vi "자판기.vi"() -> ()   [LabVIEW 2023]
panel:
  in  "커피":bool
  in  "콜라":bool
  in  "아이스티":bool
  in  "반환":bool
  out "현재 금액":i32
  in  "종료":bool
  in  "물":bool
  in  "1000":bool
  in  "500":bool
  in  "100":bool
  # "커피"
  # "물"
  # "아이스티"
  # "콜라"
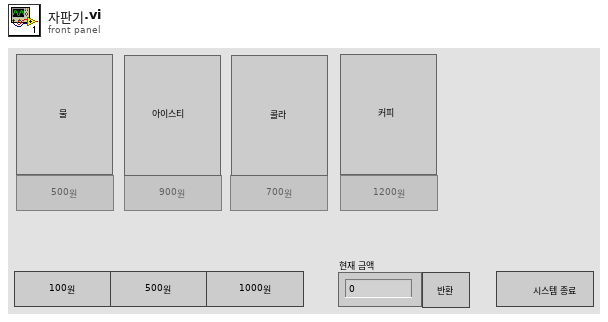
[diagram p1: front panel]
types:
  T1 = enum8{"Enabled", "Disabled", "Disabled and Grayed Out"}
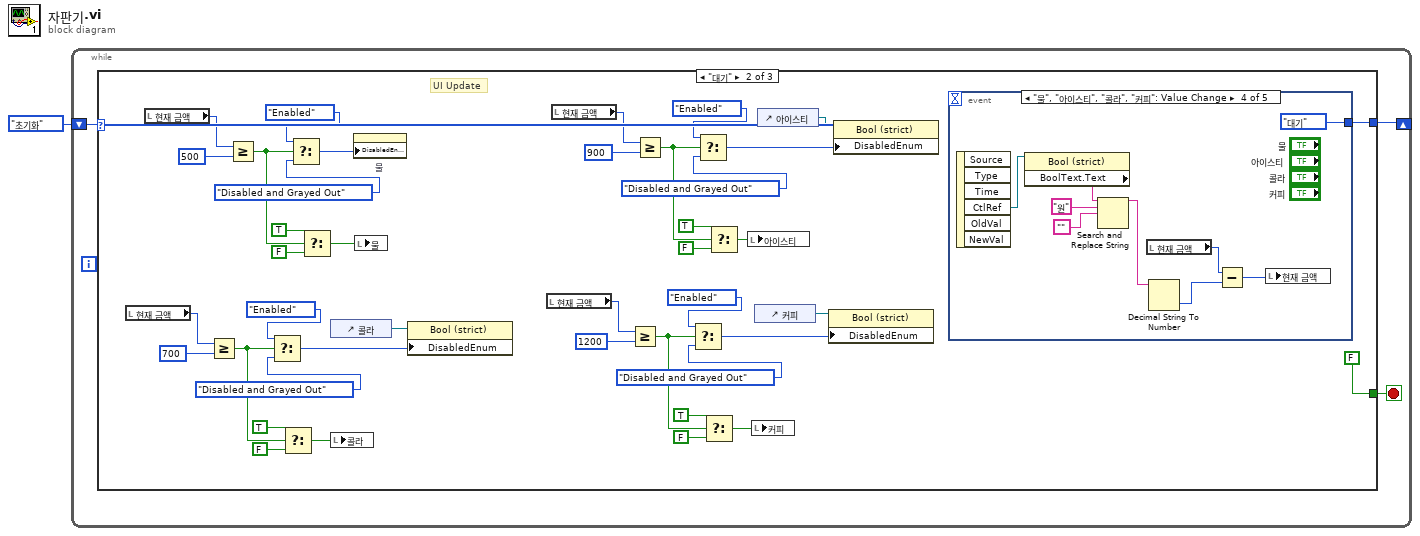
[diagram p0: block diagram]
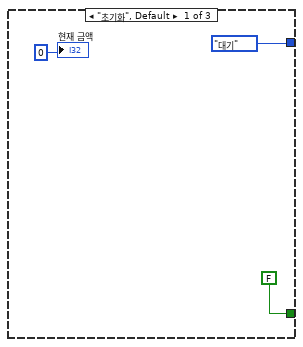
[diagram p2: hidden frame]
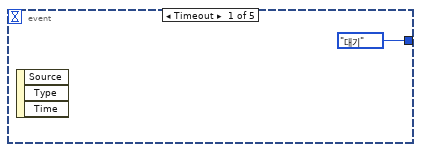
[diagram p3: hidden frame]
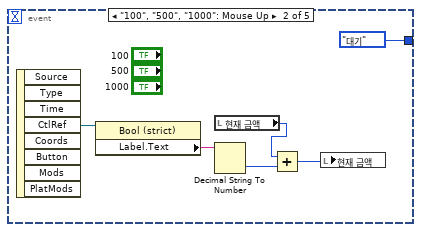
[diagram p4: hidden frame]
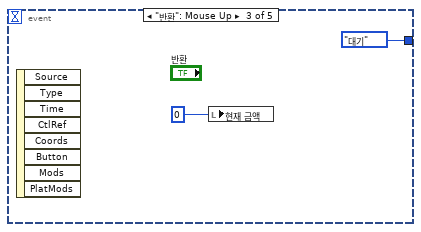
[diagram p5: hidden frame]
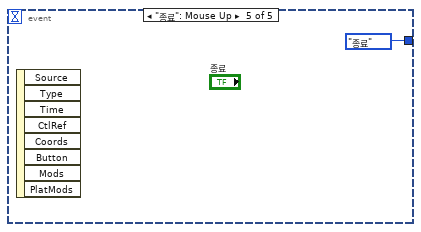
[diagram p6: hidden frame]
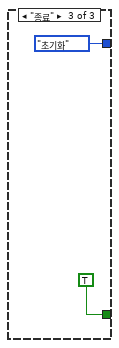
[diagram p7: hidden frame]
diagram:
  n1 = while {
    shift-right: [w3] -> _
    shift-left: enum16{"초기화", "대기", "종료"}."초기화" -> [w4]
    stop <- w2 stop-if-true
    n2 = case shown="\"대기\"" w4 {
      tunnel: [enum16{"초기화", "대기", "종료"}."대기" w48 enum16{"초기화", "대기", "종료"}."초기화"] -> w3
      tunnel: [FALSE FALSE TRUE] -> w2
      frame "초기화", Default {
        "현재 금액" <- 0 ("현재 금액")
      }
      frame "대기" {
        # "UI Update"
        n3 = local read "현재 금액"() -> (w28:i32)
        n4 = local read "현재 금액"() -> (w47:i32)
        n5 = Greater Or Equal?(x=w28, y=700) -> (x >= y?=w24:bool)
        n6 = Greater Or Equal?(x=w47, y=500) -> (x >= y?=w42:bool)
        n7 = Select(t=T1."Enabled" ("Disabled"), s=w24, f=T1."Disabled and Grayed Out" ("Disabled")) -> (s? t:f=w20:T1)
        n8 = Select(t=TRUE, s=w24, f=FALSE) -> (s? t:f=w21:bool)
        n9 = Select(t=T1."Enabled" ("Disabled"), s=w42, f=T1."Disabled and Grayed Out" ("Disabled")) -> (s? t:f=w45:T1)
        n10 = Select(t=TRUE, s=w42, f=FALSE) -> (s? t:f=w39:bool)
        n11 = control-ref of="콜라"() -> (w19:refnum<vi>)
        n12 = local write "콜라"(w21) -> ()
        n13 = property on="물" class="Bool (strict)"("DisabledEnum"=w45) -> ()  [unwired: 2 in, 2 out]
        n14 = local write "물"(w39) -> ()
        n15 = property class="Bool (strict)"(reference=w19, "DisabledEnum"=w20) -> ()  [unwired: 1 in, 2 out]
        n16 = local read "현재 금액"() -> (w18:i32)
        n17 = local read "현재 금액"() -> (w38:i32)
        n18 = Greater Or Equal?(x=w18, y=1200) -> (x >= y?=w14:bool)
        n19 = Greater Or Equal?(x=w38, y=900) -> (x >= y?=w34:bool)
        n20 = Select(t=T1."Enabled" ("Disabled"), s=w14, f=T1."Disabled and Grayed Out" ("Disabled")) -> (s? t:f=w10:T1)
        n21 = Select(t=T1."Enabled" ("Disabled"), s=w34, f=T1."Disabled and Grayed Out" ("Disabled")) -> (s? t:f=w30:T1)
        n22 = Select(t=TRUE, s=w14, f=FALSE) -> (s? t:f=w11:bool)
        n23 = Select(t=TRUE, s=w34, f=FALSE) -> (s? t:f=w31:bool)
        n24 = local write "아이스티"(w31) -> ()
        n25 = local write "커피"(w11) -> ()
        n26 = control-ref of="커피"() -> (w9:refnum<vi>)
        n27 = control-ref of="아이스티"() -> (w29:refnum<vi>)
        n28 = property class="Bool (strict)"(reference=w9, "DisabledEnum"=w10) -> ()  [unwired: 1 in, 2 out]
        n29 = property class="Bool (strict)"(reference=w29, "DisabledEnum"=w30) -> ()  [unwired: 1 in, 2 out]
        n30 = event shown="[3] \"물\", \"아이스티\", \"콜라\", \"커피\": Value Change" {
          selector: _ -> [_ _ _ _ _]
          dyn-events: _ -> [_ _ _ _ _]
          timeout: _ -> [_ _ _ _ _]
          tunnel: [enum16{"초기화", "대기", "종료"}."대기" enum16{"초기화", "대기", "종료"}."대기" enum16{"초기화", "대기", "종료"}."대기" enum16{"초기화", "대기", "종료"}."대기" enum16{"초기화", "대기", "종료"}."종료"] -> w48
          event Timeout {
            n31 = event-data() -> ()  [unwired: 1 in, 3 out]
          }
          event "100", "500", "1000": Mouse Up {
            n32 = event-data() -> ("CtlRef"=w55:refnum<vi>)  [unwired: 1 in, 7 out]
            n33 = property class="Bool (strict)"(reference=w55) -> ("Label.Text"=w54:string)  [unwired: 1 in, 2 out]
            n34 = local read "현재 금액"() -> (w52:i32)
            n35 = Decimal String To Number(string=w54) -> (number=w53:i32)  [unwired: 2 in, 1 out]
            n36 = Add(x=w52, y=w53) -> (x+y=w51:i32)
            n37 = local write "현재 금액"(w51) -> ()
          }
          event "반환": Mouse Up {
            n38 = event-data() -> ()  [unwired: 1 in, 8 out]
            n39 = local write "현재 금액"(0 ("현재 금액")) -> ()
          }
          event "물", "아이스티", "콜라", "커피": Value Change {
            n40 = event-data() -> ("CtlRef"=w63:refnum<vi>)  [unwired: 1 in, 5 out]
            n41 = property class="Bool (strict)"(reference=w63) -> ("BoolText.Text"=w61:string)  [unwired: 1 in, 2 out]
            n42 = Search and Replace String(input string=w61, search string="원", replace string="") -> (result string=w62:string)  [unwired: 5 in, 3 out]
            n43 = local read "현재 금액"() -> (w65:i32)
            n44 = Decimal String To Number(string=w62) -> (number=w58:i32)  [unwired: 2 in, 1 out]
            n45 = Subtract(x=w65, y=w58) -> (x-y=w66:i32)
            n46 = local write "현재 금액"(w66) -> ()
          }
          event "종료": Mouse Up {
            n47 = event-data() -> ()  [unwired: 1 in, 8 out]
          }
        }
      }
      frame "종료" {
      }
    }
  }
